vi "Meandr_FIFO_host.vi"() -> ()   [LabVIEW 2018]
uses:
  <vilib>/userdefined/High Color/nirio_resource_hc.ctl
  1661RR035_prog_l/FPGA Bitfiles/Code_TypeDef.ctl
  <vilib>/FPGAPlugInAG/PXI-7951R/niLvFpga_Open_PXI-7951R.vi
  <vilib>/FPGAPlugInAG/PXI-7951R/niLvFpga_Reset_PXI-7951R.vi
  <vilib>/FPGAPlugInAG/PXI-7951R/niLvFpga_Run_PXI-7951R.vi
  <vilib>/Utility/error.llb/Error Cluster From Error Code.vi
  <vilib>/rvi/errors/niLvFpgaAdjustHostInterfaceError.vi
  <vilib>/FPGAPlugInAG/PXI-7951R/niLvFpga_Close_PXI-7951R.vi
  <vilib>/rvi/interface/nirviOpenFPGA/nirviOpenFPGA.xnode
  FPGA Bitfiles/FPGAstudy_FPGATarget_MeandrFIFOtarget_r6HHcdNtsMc.lvbitx
  <vilib>/rvi/interface/nirviMethod/nirviMethod.xnode
  <vilib>/rvi/interface/nirviReadWriteControl/nirviReadWriteControl.xnode
  <vilib>/rvi/interface/nirviCloseFPGA/nirviCloseFPGA.xnode
  NiFpgaLv.dll
  <vilib>/FPGAPlugInAG/PXI-7951R/niLvFpga_WriteFifo_PXI-7951R.vi
  <vilib>/rvi/errors/niLvFpgaMergeErrorWithErrorCode.vi
panel:
  out "unsigned 8bit integer":u8 format="%b"
  in  "Mode":u16(ring)=2 items=["Code"=1, "Code On"=2, "Meandr"=3]
  in  "Code On":T1
  in  "Start number (increment/decrement) (on)":i32
  out "Empty Elements Remaining":u32=262153
  out "Push?":bool
  in  "stop":bool
  out "Pushed?":bool
  in  "Code":T1=enum."Increment+"
  in  "Start number (increment/decrement)":i32
  in  "Timeout (ms)":i32=-1
  in  "Word write":u16=255 format="%b"
  out "initialized array":u8[](array[numeric])=[255] format="%08b"
  in  "Время импульса, нс":i32=10
  in  "Скважность":i32=2
  out "error out (4110)":errorcluster
  in  "Stop Power":bool
  in  "Voltage level CH0":dbl=1.0 format="%#_13g"
  in  "Voltage level CH2":dbl=-1.0 format="%#_13g"
  in  "Voltage level CH1":dbl=3.0
  out "I CH0.0, A":dbl=0.00013065768456271712
  out "I CH0.1, A":dbl=-2.0284052519059222e-05
  out "I CH0.2, A":dbl=1.3984313200299876e-06
  in  "Current limit CH0":dbl=0.1 format="%#_13g"
  in  "Current limit CH2":dbl=0.1 format="%#_13g"
  in  "Current limit CH1":dbl=0.7 format="%#_13g"
  out "U CH0.0, В":dbl=0.0002661591678421001
  out "U CH0.1, В":dbl=2.9997050415329616
  out "U CH0.2, В":dbl=-0.0007642235631515204
  in  "Output enabled CH0":bool
  in  "Output enabled CH0 2":bool=TRUE
  in  "Output enabled CH0 3":bool
  in  "Power Resource":refnum<k15>="PXI1Slot3"
  out "error out (FPGA)":errorcluster
  in  "resource name":T2="PXI1Slot2" caption="RIO Device"
  # "Меандр"
  # "Источник питания"
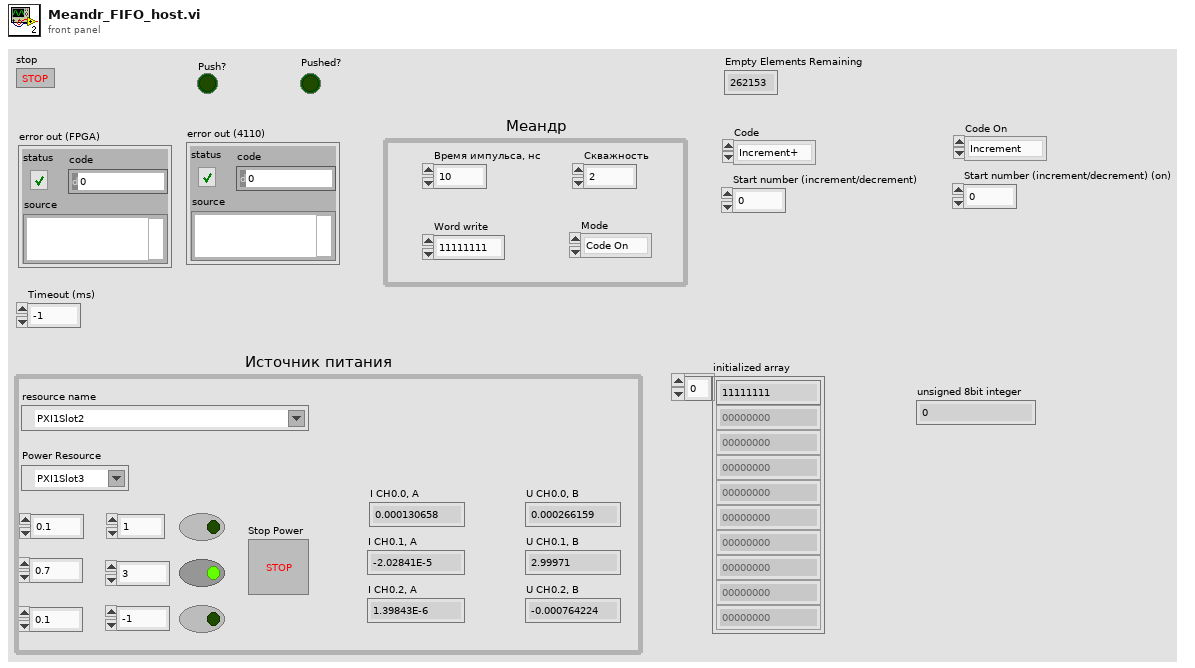
[diagram p1: front panel]
types:
  T1 = typedef "Code_TypeDef.ctl" = enum16{"Increment", "Decrement", "Chess", "NChess", "One", "Zero", "random", "Increment+", "00000001", "00000010", "00000011"}
  T2 = typedef "nirio_resource_hc.ctl" = tag
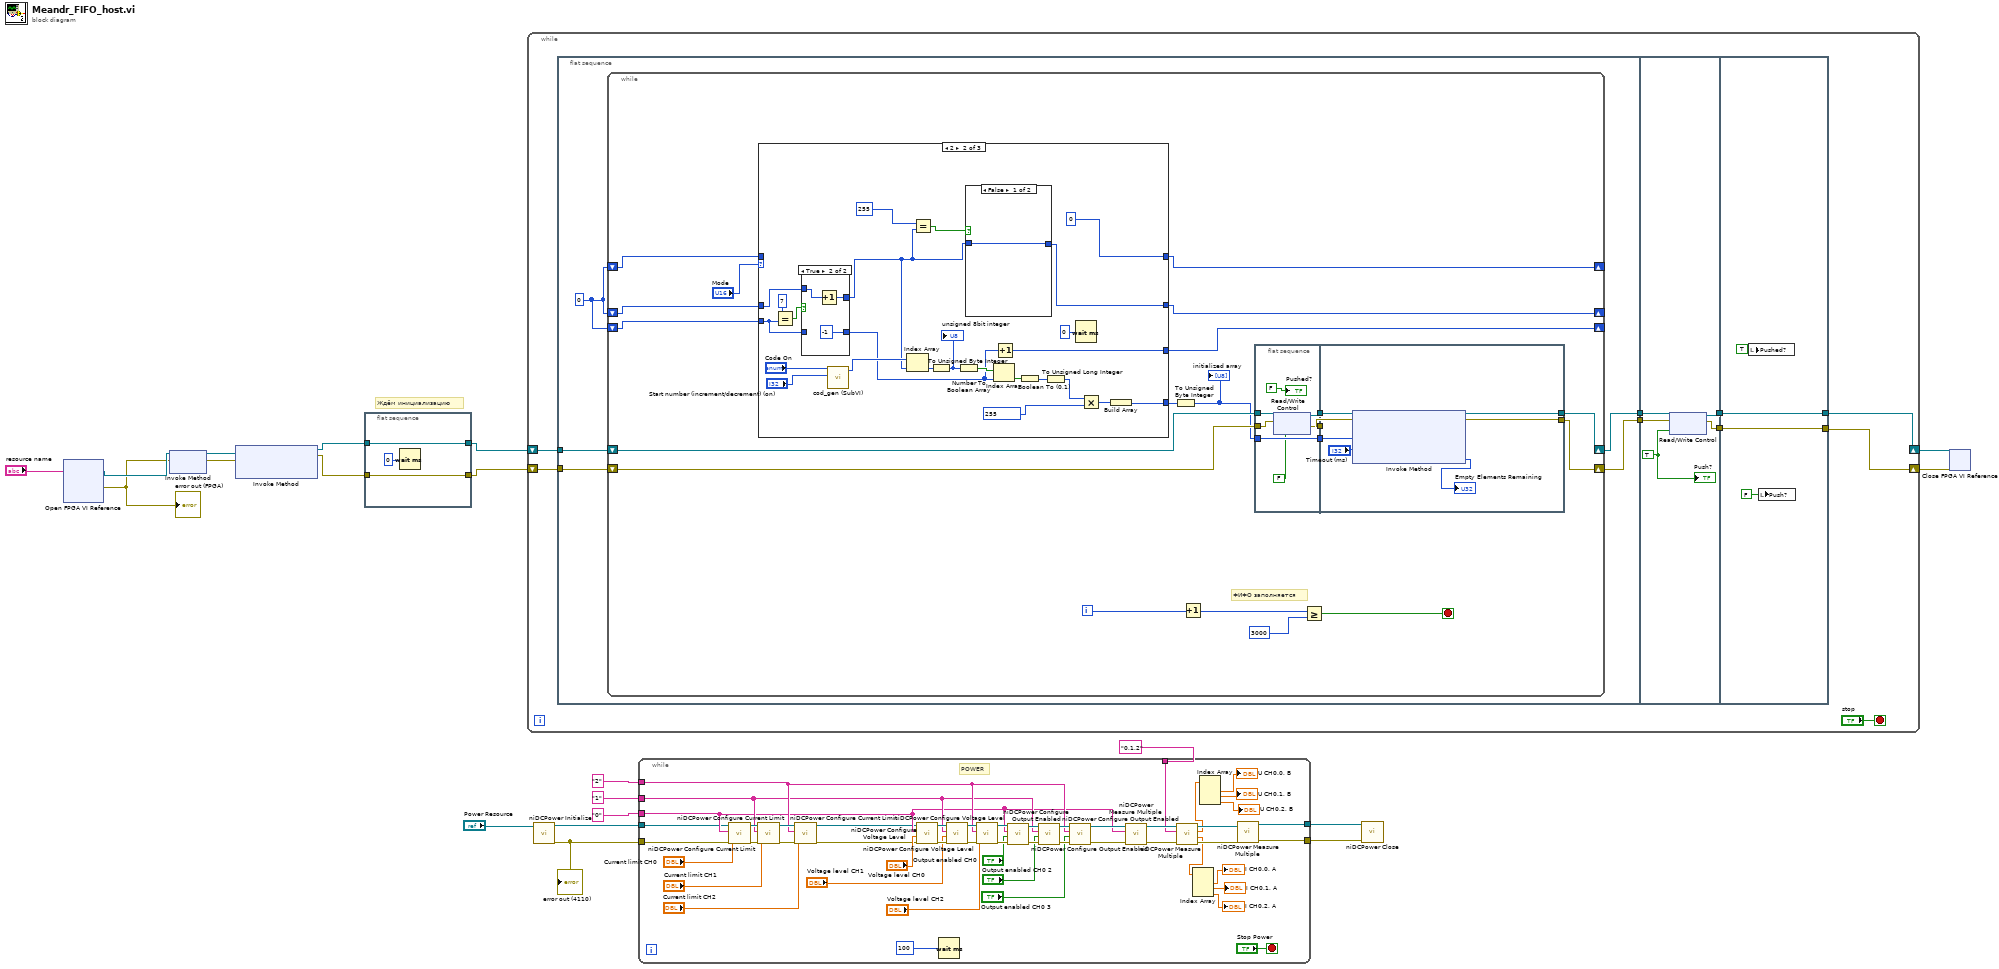
[diagram p0: block diagram]
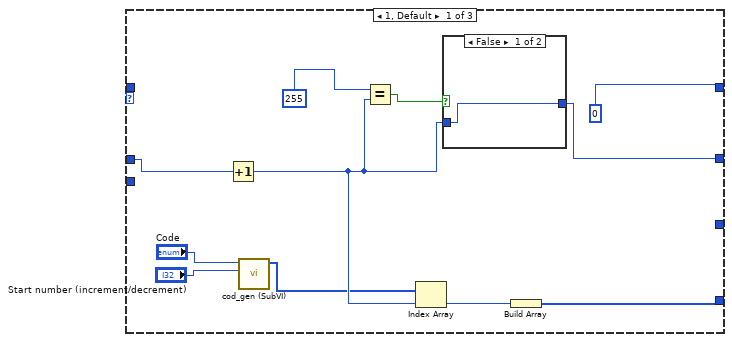
[diagram p2: hidden frame]
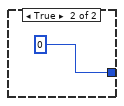
[diagram p3: hidden frame]
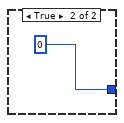
[diagram p5: hidden frame]
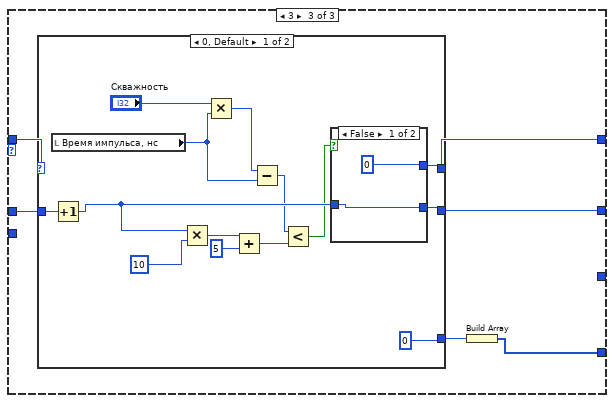
[diagram p6: hidden frame]
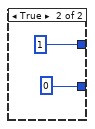
[diagram p7: hidden frame]
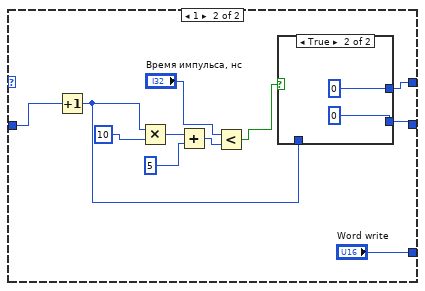
[diagram p8: hidden frame]
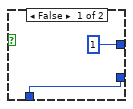
[diagram p9: hidden frame]
diagram:
  # "Ждём инициализацию"
  n1 = xnode "Open FPGA VI Reference"("resource name"="resource name") -> ("FPGA VI Reference Out"=w19:refnum<k20>, "error out"=w18:errorcluster)  [unwired: 1 in]
  "error out (FPGA)" <- w18
  n2 = xnode "Invoke Method"("FPGA VI Reference In"=w19, "error in"=w18) -> ("FPGA VI Reference Out"=w8:refnum<k20>, "error out"=w17:errorcluster)
  n3 = xnode ("Invoke Method")("FPGA VI Reference In"=w8, "error in"=w17) -> ("FPGA VI Reference Out"=w7:refnum<k20>, "error out"=w6:errorcluster)  [unwired: 1 in]
  n4 = flat-sequence {
    tunnel: [w22] -> w1
    tunnel: w7 -> [w22]
    tunnel: [w21] -> w2
    tunnel: w6 -> [w21]
    frame #0 {
      n5 = Wait (ms)(milliseconds to wait=u32 0) -> ()  [unwired: 1 out]
    }
  }
  n6 = while {
    shift-right: [w29] -> w4
    shift-left: w2 -> [w32]
    shift-right: [w30] -> w5
    shift-left: w1 -> [w31]
    stop <- "stop" stop-if-true
    n7 = flat-sequence {
      tunnel: w32 -> [w37]
      tunnel: w31 -> [w36]
      tunnel: [w35] -> w27
      tunnel: [w34] -> w26
      tunnel: w27 -> [w158]
      tunnel: w26 -> [w157]
      tunnel: [w156] -> w25
      tunnel: [w155] -> w24
      tunnel: w25 -> [w161]
      tunnel: w24 -> [w160]
      tunnel: [w161] -> w30
      tunnel: [w160] -> w29
      frame #0 {
        w33 = 0
        n8 = while {
          shift-right: [w47] -> w34
          shift-left: w37 -> [w53]
          shift-right: [w48] -> w35
          shift-left: w36 -> [w52]
          shift-right: [w54] -> _
          shift-left: w33 -> [w57]
          shift-right: [w55] -> _
          shift-left: w33 -> [w56]
          shift-right: [w38] -> _
          shift-left: w33 -> [w39]
          i -> [w46]
          stop <- w41 stop-if-true
          # "ФИФО заполняется"
          n9 = case shown="2" "Mode" {
            tunnel: w57 -> [w81 w89 w121]
            tunnel: w56 -> [_ _ w120]
            tunnel: [0 0 w119] -> w55
            tunnel: [w78 w102 w118] -> w54
            tunnel: [w73 w99 w117] -> w42
            tunnel: w39 -> [_ w92 _]
            tunnel: [_ w94 _] -> w38
            frame 1, Default {
              n10 = Increment(x=w81) -> (x+1=w77:i32)
              n11 = call "cod_gen (SubVI).vi"("Numeric"="Start number (increment/decrement)", "Code"="Code") -> ("Array"=w72:u16[])  [unwired: 9 in]
              n12 = Equal?(x=255, y=w77) -> (x = y?=w79:bool)
              n13 = Index Array(array=w72, index=w77) -> (element=w76:u16)
              n14 = case shown="False" w79 {
                tunnel: [w83 0] -> w78
                tunnel: w77 -> [w83 _]
                frame False {
                }
                frame True {
                }
              }
              n15 = Build Array(w76) -> (w73:u16[])
            }
            frame 2 {
              n16 = Equal?(x=7, y=w92) -> (x = y?=w90:bool)
              n17 = case shown="True" w90 {
                tunnel: [w110 -1] -> w93
                tunnel: w92 -> [w110 _]
                tunnel: w89 -> [w109 w112]
                tunnel: [w109 w111] -> w88
                frame False {
                }
                frame True {
                  n18 = Increment(x=w112) -> (x+1=w111:i32)
                }
              }
              n19 = call "cod_gen (SubVI).vi"("Numeric"="Start number (increment/decrement) (on)", "Code"="Code On") -> ("Array"=w104:u16[])  [unwired: 9 in]
              n20 = Index Array(array=w104, index=w88) -> (element=w85:u16)
              n21 = Equal?(x=255, y=w88) -> (x = y?=w107:bool)
              n22 = To Unsigned Byte Integer(number=w85) -> (unsigned 8bit integer=w86:u8)
              "unsigned 8bit integer" <- w86
              n23 = Number To Boolean Array(number=w86) -> (Boolean array=w101:bool[])
              n24 = case shown="False" w107 {
                tunnel: [w114 0] -> w102
                tunnel: w88 -> [w114 _]
                frame False {
                }
                frame True {
                }
              }
              n25 = Index Array(array=w101, index=w93) -> (element=w100:bool)
              n26 = Increment(x=w93) -> (x+1=w94:i32)
              n27 = Boolean To (0,1)(Boolean=w100) -> (0, 1=w96:i16)
              n28 = To Unsigned Long Integer(number=w96) -> (unsigned 32bit integer=w95:u32)
              n29 = Wait (ms)(milliseconds to wait=u32 0) -> ()  [unwired: 1 out]
              n30 = Multiply(x=w95, y=u32 255) -> (x*y=w98:u32)
              n31 = Build Array(w98) -> (w99:u32[])
            }
            frame 3 {
              n32 = case shown="0, Default" w120 {
                tunnel: [w135 w150] -> w119
                tunnel: [w133 w149] -> w118
                tunnel: [u16 0 "Word write"] -> w116
                tunnel: w121 -> [w132 w148]
                frame 0, Default {
                  n33 = local read "Время импульса, нс"() -> (w129:i32)
                  n34 = Increment(x=w132) -> (x+1=w128:i32)
                  n35 = Multiply(x=w128, y=10) -> (x*y=w126:i32)
                  n36 = Multiply(x="Скважность", y=w129) -> (x*y=w130:i32)
                  n37 = Add(x=w126, y=5) -> (x+y=w122:i32)
                  n38 = Subtract(x=w130, y=w129) -> (x-y=w123:i32)
                  n39 = Less?(x=w123, y=w122) -> (x < y?=w124:bool)
                  n40 = case shown="False" w124 {
                    tunnel: [0 1] -> w135
                    tunnel: [w136 0] -> w133
                    tunnel: w128 -> [w136 _]
                    frame False {
                    }
                    frame True {
                    }
                  }
                }
                frame 1 {
                  n41 = Increment(x=w148) -> (x+1=w145:i32)
                  n42 = Multiply(x=w145, y=10) -> (x*y=w144:i32)
                  n43 = Add(x=w144, y=5) -> (x+y=w140:i32)
                  n44 = Less?(x="Время импульса, нс", y=w140) -> (x < y?=w142:bool)
                  n45 = case shown="True" w142 {
                    tunnel: [1 0] -> w150
                    tunnel: w145 -> [w151 _]
                    tunnel: [w151 0] -> w149
                    frame False {
                    }
                    frame True {
                    }
                  }
                }
              }
              n46 = Build Array(w116) -> (w117:u16[])
            }
          }
          n47 = To Unsigned Byte Integer(number=w42) -> (unsigned 8bit integer=w43:u8[])
          "initialized array" <- w43
          n48 = Increment(x=w46) -> (x+1=w45:i32)
          n49 = flat-sequence {
            tunnel: w52 -> [w61]
            tunnel: w53 -> [w60]
            tunnel: w43 -> [w64]
            tunnel: [w64] -> w51
            tunnel: [w62] -> w50
            tunnel: [w63] -> w49
            tunnel: w51 -> [w71]
            tunnel: w50 -> [w69]
            tunnel: w49 -> [w68]
            tunnel: [w67] -> w48
            tunnel: [w66] -> w47
            frame #0 {
              n50 = xnode "Read/Write Control"("FPGA VI Reference In"=w61, "error in"=w60, "Push?"=FALSE) -> ("FPGA VI Reference Out"=w63:refnum<k20>, "error out"=w62:errorcluster)
              "Pushed?" <- FALSE
            }
            frame #1 {
              n51 = xnode "Invoke Method"("FPGA VI Reference In"=w68, "error in"=w69, "Data"=w71, "Timeout (ms)"="Timeout (ms)") -> ("FPGA VI Reference Out"=w67:refnum<k20>, "error out"=w66:errorcluster, "Empty Elements Remaining"=→"Empty Elements Remaining":u32)
            }
          }
          n52 = Greater Or Equal?(x=w45, y=3000) -> (x >= y?=w41:bool)
        }
      }
      frame #1 {
        w159 = TRUE ("Push?")
        n53 = xnode "Read/Write Control"("FPGA VI Reference In"=w158, "error in"=w157, "Push?"=w159) -> ("FPGA VI Reference Out"=w156:refnum<k20>, "error out"=w155:errorcluster)
        "Push?" <- w159
      }
      frame #2 {
        n54 = local write "Pushed?"(TRUE ("Pushed?")) -> ()
        n55 = local write "Push?"(FALSE ("Push?")) -> ()
      }
    }
  }
  n56 = call <instrlib>:"niDCPower Initialize.vi"("resource name"="Power Resource") -> ("error out"=w9:errorcluster, "instrument handle out"=w10:refnum<k15>)  [unwired: 3 in, 6 out]
  "error out (4110)" <- w9
  n57 = while {
    tunnel: "0" ("Channel name") -> [w175]
    tunnel: [w192] -> w15
    tunnel: [w195] -> w14
    tunnel: "1" -> [w177]
    tunnel: "2" -> [w178]
    tunnel: w9 -> [w176]
    tunnel: w10 -> [w174]
    tunnel: "0,1,2" ("channel name") -> [w164]
    stop <- "Stop Power" stop-if-true
    # "POWER"
    n58 = call <instrlib>:"niDCPower Configure Current Limit.vi"("error in (no error)"=w176, "current limit"="Current limit CH0", "channel name"=w175, "instrument handle"=w174) -> ("error out"=w182:errorcluster, "instrument handle out"=w180:refnum<k15>)  [unwired: 6 in]
    n59 = call <instrlib>:"niDCPower Configure Current Limit.vi"("error in (no error)"=w182, "current limit"="Current limit CH1", "channel name"=w177, "instrument handle"=w180) -> ("error out"=w183:errorcluster, "instrument handle out"=w181:refnum<k15>)  [unwired: 6 in]
    n60 = call <instrlib>:"niDCPower Configure Current Limit.vi"("error in (no error)"=w183, "current limit"="Current limit CH2", "channel name"=w178, "instrument handle"=w181) -> ("error out"=w173:errorcluster, "instrument handle out"=w172:refnum<k15>)  [unwired: 6 in]
    n61 = call <instrlib>:"niDCPower Configure Voltage Level.vi"("error in (no error)"=w173, "voltage level"="Voltage level CH0", "channel name"=w175, "instrument handle"=w172) -> ("error out"=w209:errorcluster, "instrument handle out"=w205:refnum<k15>)  [unwired: 6 in]
    n62 = Wait (ms)(milliseconds to wait=u32 100) -> ()  [unwired: 1 out]
    n63 = call <instrlib>:"niDCPower Configure Voltage Level.vi"("error in (no error)"=w209, "voltage level"="Voltage level CH1", "channel name"=w177, "instrument handle"=w205) -> ("error out"=w208:errorcluster, "instrument handle out"=w204:refnum<k15>)  [unwired: 6 in]
    n64 = call <instrlib>:"niDCPower Configure Voltage Level.vi"("error in (no error)"=w208, "voltage level"="Voltage level CH2", "channel name"=w178, "instrument handle"=w204) -> ("error out"=w207:errorcluster, "instrument handle out"=w206:refnum<k15>)  [unwired: 6 in]
    n65 = call <instrlib>:"niDCPower Configure Output Enabled.vi"("error in (no error)"=w207, "output enabled"="Output enabled CH0", "channel name"=w175, "instrument handle"=w206) -> ("error out"=w202:errorcluster, "instrument handle out"=w203:refnum<k15>)  [unwired: 6 in]
    n66 = call <instrlib>:"niDCPower Configure Output Enabled.vi"("error in (no error)"=w202, "output enabled"="Output enabled CH0 2", "channel name"=w177, "instrument handle"=w203) -> ("error out"=w201:errorcluster, "instrument handle out"=w200:refnum<k15>)  [unwired: 6 in]
    n67 = call <instrlib>:"niDCPower Configure Output Enabled.vi"("error in (no error)"=w201, "output enabled"="Output enabled CH0 3", "channel name"=w178, "instrument handle"=w200) -> ("error out"=w198:errorcluster, "instrument handle out"=w199:refnum<k15>)  [unwired: 6 in]
    n68 = call <instrlib>:"niDCPower Measure Multiple.vi"("error in (no error)"=w198, "channel name"=w175, "instrument handle"=w199) -> ("error out"=w194:errorcluster, "instrument handle out"=w197:refnum<k15>)  [unwired: 5 in, 2 out]
    n69 = call <instrlib>:"niDCPower Measure Multiple.vi"("error in (no error)"=w194, "channel name"=w164, "instrument handle"=w197) -> ("error out"=w193:errorcluster, "current measurements"=w189:dbl[], "voltage measurements"=w171:dbl[], "instrument handle out"=w196:refnum<k15>)  [unwired: 5 in]
    n70 = Index Array(array=w189) -> (element #1=→"I CH0.0, A":dbl, element #2=→"I CH0.1, A":dbl, element #3=→"I CH0.2, A":dbl)  [unwired: 3 in]
    n71 = Index Array(array=w171) -> (element #1=→"U CH0.0, В":dbl, element #2=→"U CH0.1, В":dbl, element #3=→"U CH0.2, В":dbl)  [unwired: 3 in]
    n72 = call <instrlib>:"niDCPower Measure Multiple.vi"("error in (no error)"=w193, "instrument handle"=w196) -> ("error out"=w192:errorcluster, "instrument handle out"=w195:refnum<k15>)  [unwired: 6 in, 2 out]
  }
  n73 = call <instrlib>:"niDCPower Close.vi"("error in (no error)"=w15, "instrument handle"=w14) -> ()  [unwired: 9 in, 1 out]
  n74 = xnode "Close FPGA VI Reference"("FPGA VI Reference In"=w5, "error in"=w4) -> ()  [unwired: 1 out]
